vi "PXDAC4800_SetOutputVoltageCh2XD48.vi"(2 "Value":u32, 3 "Handle":u32) -> (0 "Status":i32, 1 "Handle out":u32)   [LabVIEW 2016]
uses:
  PXDAC4800.dll
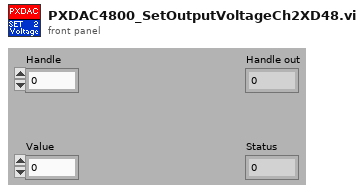
[diagram p1: front panel]
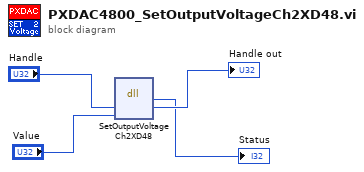
[diagram p0: block diagram]
diagram:
  n1 = dll-call lib="PXDAC4800.dll" fn="SetOutputVoltageCh2XD48"("Handle"="Handle", "Val"="Value") -> (→"Status":i32, "Handle"=→"Handle out":u32)  [unwired: 4 in, 2 out]
